vi "PrepareHWI.vi"(8 "error in (no error)":errorcluster, 9 "Master Device.lvclass":refnum<class "Master Device.lvclass">, 10 "Current Variables":T1[](array[typedef]), 11 "Pulseblaster in":refnum<class "Pulseblaster.lvclass">) -> (0 "error out":errorcluster, 2 "Master Device out":refnum<class "Master Device.lvclass">, 3 "Pulseblaster out":refnum<class "Pulseblaster.lvclass">)   [LabVIEW 2013, in "Pulseblaster.lvclass"]
uses:
  Pulseblaster.lvclass
  TypeDefs/Active procedure variables.ctl
  Master Device/Master Device.lvclass
  TypeDefs/RampInfo.ctl
  TypeDefs/SlaveInfo.ctl
  Pulseblaster.lvclass/Pulseblaster.ctl
  Utils_devs/PB_HWI/PulseBlaster.lvlib
panel:
  out "parsed t":dbl format="%#_15g"
  out "parsed dt":dbl format="%#_15g"
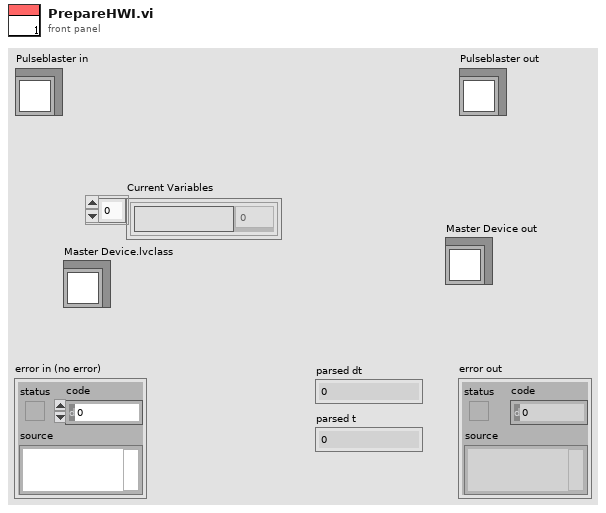
[diagram p1: front panel]
types:
  T1 = typedef "Active procedure variables.ctl" = cluster{"Procedure variable":string, "Value":dbl}
  T2 = typedef "SlaveInfo.ctl" = cluster{"Triggering":bool[][], "Ramp Info":T3[], "Line Inversion":bool[], "Slaved Digital Channels":cluster{"Master Channel Number":i32, "Output States":bool[]}[]}
  T3 = typedef "RampInfo.ctl" = cluster{"Table Ramp Index":i32, "Ramp Time":dbl, "Number of Steps":i32, "Instruction Array Index":i32}
  T4 = cluster{"Output Bits":u32, "Data Field":u32, "OP Code":u8, "Delay Count":u64}[]
  T5 = cluster{"External MemorySize":u16, "Internal Memory Size":u16, "Overhead Ticks":u8, "Min Delay Loops":u8, "Loop Count Correction":u8, "Long Delay Loop Count Correction":u8, "Min Instruction Ticks":u8, "Long Delay Ticks":u64, "Clock Period (s)":dbl, "Overhead Time (s)":dbl, "Min Instruction Cycle Time (s)":dbl, "Long Delay Time (s) ":dbl}
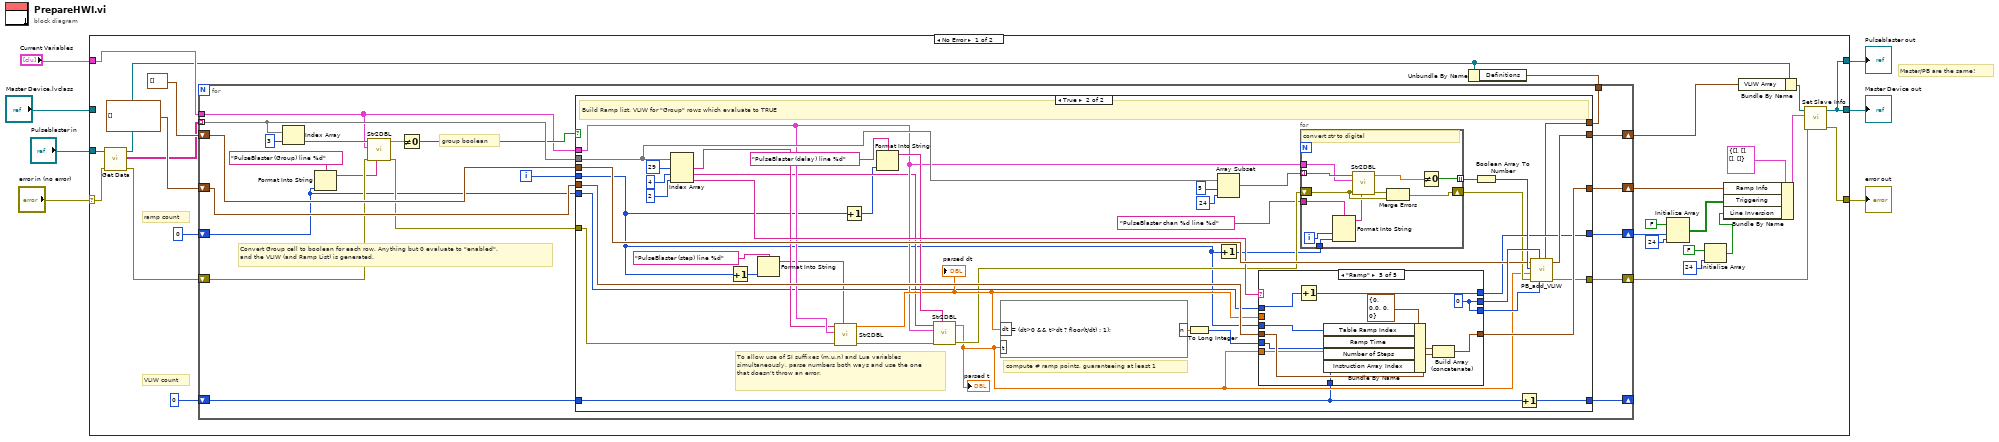
[diagram p0: block diagram]
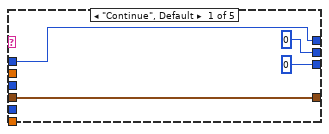
[diagram p3: hidden frame]
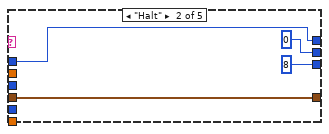
[diagram p4: hidden frame]
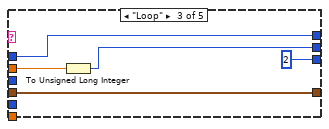
[diagram p5: hidden frame]
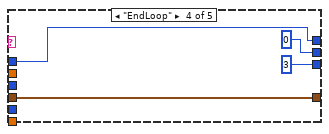
[diagram p6: hidden frame]
diagram:
  # "Master/PB are the same!"
  n1 = case shown="No Error" "error in (no error)" {
    selector: "error in (no error)" -> [w22 w141]
    tunnel: [w12 w141] -> w5
    tunnel: "Pulseblaster in" -> [w23 w143]
    tunnel: [w11 w143] -> w7
    tunnel: "Master Device.lvclass" -> [_ w142]
    tunnel: "Current Variables" -> [w33 _]
    tunnel: [w11 w142] -> w4
    frame No Error {
      # "VLIW count"
      # "ramp count"
      n2 = call-dynamic "Get Data.vi"("error in (no error)"=w22, "Device in"=w23) -> ("error out"=w32:errorcluster, "Table Indicator"=w27:string[][], "Device out"=w21:refnum<class "Pulseblaster.lvclass">)  [unwired: 6 in]
      n3 = Unbundle By Name(w21) -> ("Definitions"=w20:T5)
      n4 = for {
        tunnel: w27 -> [w48] mode=indexing
        tunnel: w33 -> [w41]
        shift-right: [w51] -> w13
        shift-left: w32 -> [w45]
        shift-right: [w50] -> w24
        shift-left: T4 [] ("VLIW Array In") -> [w54]
        shift-right: [w52] -> w16
        shift-left: T3[] [] -> [w53]
        shift-right: [w49] -> w25
        shift-left: 0 -> [w40]
        tunnel: w20 -> [w36]
        shift-right: [w34] -> _
        shift-left: 0 -> [w35]
        i -> [w37]
        # "group boolean"
        # "Convert Group cell to boolean for each row. Anything but 0 evaluate to \"enabled\",\nand the VLIW (and Ramp List) is generated."
        n5 = Index Array(array=w48, index=3) -> (element=w46:string)
        n6 = Format Into String(format string="PulseBlaster (Group) line %d", w40) -> (resulting string=w38:string)  [unwired: 2 in, 1 out]
        n7 = call "Str2DBL.vi"("Error Locator"=w38, "error in (no error)"=w45, "Current Variable settings"=w41, "formula"=w46) -> ("error out"=w44:errorcluster, "y value"=w43:dbl)  [unwired: 4 in]
        n8 = Not Equal To 0?(x=w43) -> (x != 0?=w42:bool)
        n9 = case shown="True" w42 {
          tunnel: w44 -> [w56 w69]
          tunnel: w41 -> [_ w77]
          tunnel: w48 -> [_ w93]
          tunnel: w54 -> [w57 w92]
          tunnel: w53 -> [w58 w88]
          tunnel: w37 -> [_ w66]
          tunnel: [w58 w87] -> w52
          tunnel: [w56 w86] -> w51
          tunnel: [w57 w85] -> w50
          tunnel: w40 -> [w59 w74]
          tunnel: [w59 w84] -> w49
          tunnel: w36 -> [_ w62]
          tunnel: w35 -> [w55 w60]
          tunnel: [w55 w61] -> w34
          frame False {
          }
          frame True {
            # "compute # ramp points, guaranteeing at least 1"
            # "To allow use of SI suffixes (m,u,n) and Lua variables simultaneously, parse numbers both ways and use the one that doesn't throw an error."
            # "Build Ramp list, VLIW for \"Group\" rows which evaluate to TRUE"
            n10 = Index Array(array=w93, index #1=29 ("index"), index #2=4 ("index"), index #3=2 ("index")) -> (element #1=w76:string, element #2=w71:string, element #3=w83:string)
            n11 = Increment(x=w66) -> (x+1=w67:i32)
            n12 = Format Into String(format string="PulseBlaster (step) line %d", w67) -> (resulting string=w72:string)  [unwired: 2 in, 1 out]
            n13 = call "Str2DBL.vi"("Error Locator"=w72, "error in (no error)"=w69, "Current Variable settings"=w77, "formula"=w76) -> ("error out"=w75:errorcluster, "y value"=w78:dbl)  [unwired: 4 in]
            "parsed dt" <- w78
            n14 = Increment(x=w66) -> (x+1=w68:i32)
            n15 = Format Into String(format string="PulseBlaster (delay) line %d", w68) -> (resulting string=w80:string)  [unwired: 2 in, 1 out]
            n16 = call "Str2DBL.vi"("Error Locator"=w80, "error in (no error)"=w75, "Current Variable settings"=w77, "formula"=w71) -> ("error out"=w70:errorcluster, "y value"=w63:dbl)  [unwired: 4 in]
            "parsed t" <- w63
            n17 = formula code="n= (dt>0 && t>dt ? floor(t/dt) : 1);"("dt"=w78, "t"=w63) -> ("n"=w82:dbl)
            n18 = To Long Integer(number=w82) -> (32bit integer=w81:i32)
            n19 = Array Subset(array=w93, index=5, length=24) -> (w99:string[])
            n20 = Increment(x=w66) -> (x+1=w64:i32)
            n21 = case shown="\"Ramp\"" w83 {
              tunnel: [u8 0 u8 8 u8 2 u8 3 w140] -> w95
              tunnel: [u32 0 u32 0 w121 u32 0 w140] -> w96
              tunnel: w78 -> [_ _ w122 _ _]
              tunnel: w88 -> [w114 w118 w124 w127 w139]
              tunnel: w66 -> [_ _ _ _ w137]
              tunnel: [w114 w118 w124 w127 w138] -> w87
              tunnel: w63 -> [_ _ _ _ w136]
              tunnel: w81 -> [_ _ _ _ w135]
              tunnel: [w113 w117 w123 w126 w132] -> w84
              tunnel: w74 -> [w113 w117 w123 w126 w133]
              tunnel: w60 -> [_ _ _ _ w130]
              frame "Continue", Default {
              }
              frame "Halt" {
              }
              frame "Loop" {
                n22 = To Unsigned Long Integer(number=w122) -> (unsigned 32bit integer=w121:u32)
              }
              frame "EndLoop" {
              }
              frame "Ramp" {
                w140 = 0
                n23 = Increment(x=w133) -> (x+1=w132:i32)
                n24 = Bundle By Name(cluster=T3 {"Table Ramp Index"=0, "Ramp Time"=0.0, "Number of Steps"=0, "Instruction Array Index"=0} ("Cluster"), "Table Ramp Index"=w137, "Ramp Time"=w136, "Number of Steps"=w135, "Instruction Array Index"=w130) -> (w134:T3)
                n25 = Build Array (concatenate)(w134, w139) -> (w138:T3[])
              }
            }
            n26 = for {
              tunnel: w99 -> [w112] mode=indexing
              tunnel: [w111] -> w90 mode=indexing
              tunnel: w77 -> [w110]
              shift-right: [w103] -> w79
              shift-left: w70 -> [w105]
              tunnel: "PulseBlaster chan %d line %d" -> [w106]
              tunnel: w64 -> [w107]
              i -> [w108]
              # "convert str to digital"
              n27 = Format Into String(format string=w106, w108, w107) -> (resulting string=w102:string)  [unwired: 2 in, 1 out]
              n28 = call "Str2DBL.vi"("Error Locator"=w102, "error in (no error)"=w105, "Current Variable settings"=w110, "formula"=w112) -> ("error out"=w104:errorcluster, "y value"=w109:dbl)  [unwired: 4 in]
              n29 = Merge Errors(w104, w105) -> (w103:errorcluster)
              n30 = Not Equal To 0?(x=w109) -> (x != 0?=w111:bool)
            }
            n31 = Boolean Array To Number(Boolean array=w90) -> (number=w94:u32)
            n32 = Increment(x=w60) -> (x+1=w61:i32)
            n33 = call "PB_add_VLIW.vi"("Definitions"=w62, "OP code"=w95, "Data Field"=w96, "error in (no error)"=w79, "Delay"=w63, "Digital Bits"=w94, "VLIW Array In"=w92) -> ("error out"=w86:errorcluster, "VLIW Array Out"=w85:T4)  [unwired: 2 in, 1 out]
          }
        }
      }
      n34 = Initialize Array(FALSE, w25, 24 ("dimension size")) -> (w17:bool[][])
      n35 = Initialize Array(FALSE, 24 ("dimension size")) -> (w9:bool[])
      n36 = Bundle By Name(cluster=T2 {"Triggering"=[], "Ramp Info"=[], "Line Inversion"=[], "Slaved Digital Channels"=[]} ("Slave Info"), "Ramp Info"=w16, "Triggering"=w17, "Line Inversion"=w9) -> (w15:T2)
      n37 = Bundle By Name(cluster=w21, "VLIW Array"=w24) -> (w14:refnum<class "Pulseblaster.lvclass">)
      n38 = call-dynamic "Set Slave Info.vi"("error in (no error)"=w13, "Slave Info"=w15, "Master Device in"=w14) -> ("error out"=w12:errorcluster, "Master Device out"=w11:refnum<class "Pulseblaster.lvclass">)  [unwired: 7 in]
    }
    frame Error {
    }
  }
  "error out" <- w5
  "Pulseblaster out" <- w7
  "Master Device out" <- w4
